vi "Check_Game_Over.vi"(10 "inputArray":bool[][](array[boolean])) -> (2 "gameOver":bool)   [LabVIEW 2015]
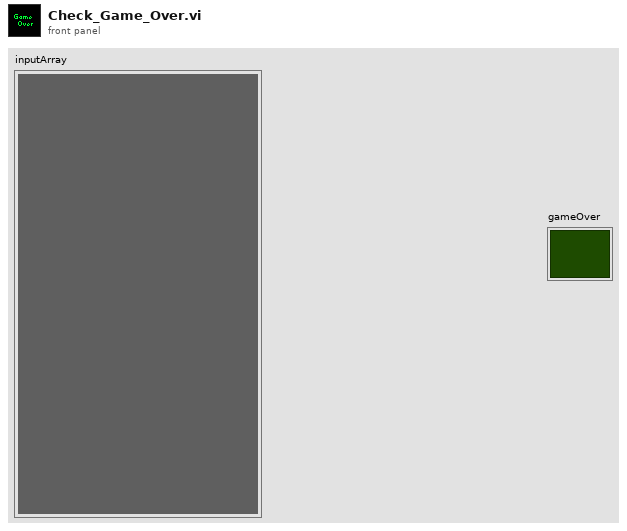
[diagram p1: front panel]
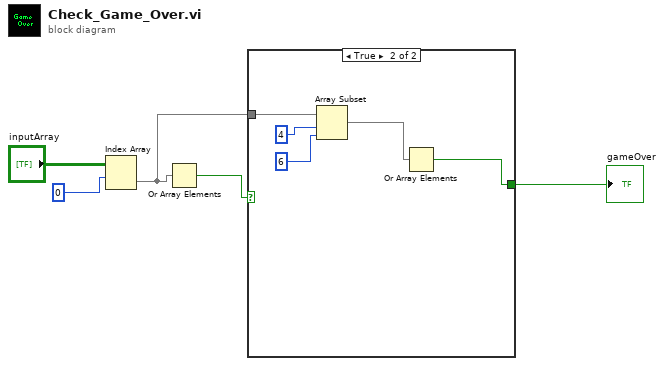
[diagram p0: block diagram]
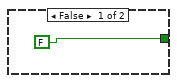
[diagram p2: hidden frame]
diagram:
  n1 = Index Array(array="inputArray", index (row)=0) -> (element=w1:bool[])  [unwired: 1 in]
  n2 = Or Array Elements(Boolean array=w1) -> (logical OR=w3:bool)
  n3 = case shown="True" w3 {
    tunnel: [FALSE w8] -> w2
    tunnel: w1 -> [_ w11]
    frame False {
    }
    frame True {
      n4 = Array Subset(array=w11, index=4, length=6) -> (w7:bool[])
      n5 = Or Array Elements(Boolean array=w7) -> (logical OR=w8:bool)
    }
  }
  "gameOver" <- w2
